vi "DisableMultiple.vi"(6 "return immediately":bool, 8 "error in (no error)":errorcluster, 10 "axis names":string[](array[string]), 11 "controller in":refnum<k24>) -> (0 "error out":errorcluster, 3 "controller out":refnum<k24>)   [LabVIEW 2020]
uses:
  C:/GEECS/Developers Version/source/Device Drivers/AerotechStage/Sample Vis/Bin/Aerotech.Ensemble.dll
  Sample Vis/Bin/Aerotech.Ensemble.dll
  C:/GEECS/Developers Version/source/Device Drivers/AerotechStage/Sample Vis/Bin/Aerotech.Ensemble.LabVIEW.dll
  Sample Vis/Bin/Aerotech.Ensemble.LabVIEW.dll
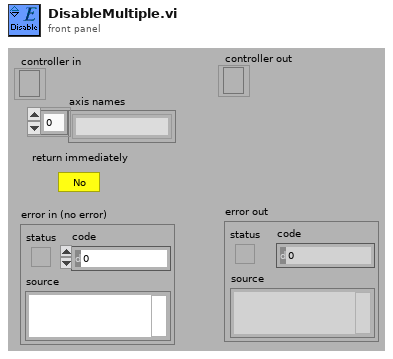
[diagram p1: front panel]
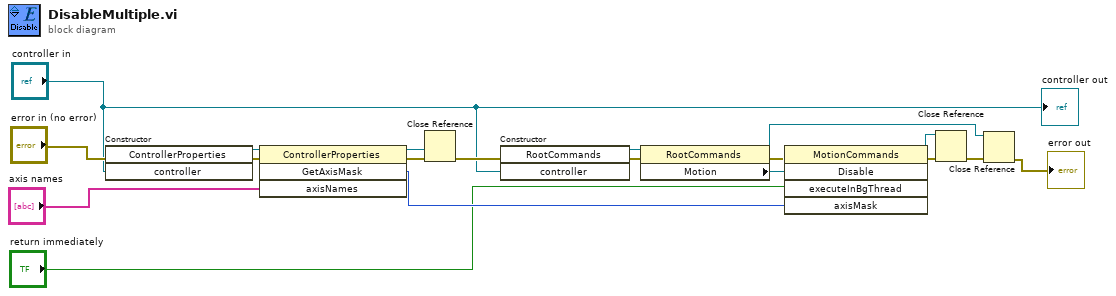
[diagram p0: block diagram]
diagram:
  n1 = constructor class="ControllerProperties"(error in="error in (no error)", "controller"="controller in") -> (reference out=w18:refnum<k24>, error out=w17:errorcluster)  [unwired: 2 in, 2 out]
  n2 = invoke class="ControllerProperties" method="GetAxisMask"(reference=w18, error in=w17, "axisNames"="axis names") -> (reference out=w15:refnum<k24>, error out=w16:errorcluster, "GetAxisMask"=w14:i32)  [unwired: 1 in, 1 out]
  n3 = Close Reference(reference=w15, error in (no error)=w16) -> (error out=w10:errorcluster)
  n4 = constructor class="RootCommands"(error in=w10, "controller"="controller in") -> (reference out=w6:refnum<k24>, error out=w5:errorcluster)  [unwired: 2 in, 2 out]
  n5 = property class="RootCommands"(reference=w6, error in=w5) -> (reference out=w1:refnum<k24>, error out=w7:errorcluster, "Motion"=w8:refnum<k24>)
  n6 = invoke class="MotionCommands" method="Disable"(reference=w8, error in=w7, "executeInBgThread"="return immediately", "axisMask"=w14) -> (reference out=w3:refnum<k24>, error out=w4:errorcluster)  [unwired: 1 in, 3 out]
  n7 = Close Reference(reference=w3, error in (no error)=w4) -> (error out=w2:errorcluster)
  n8 = Close Reference(reference=w1, error in (no error)=w2) -> (error out=→"error out":errorcluster)
  "controller out" <- "controller in"
